vi "HV Rampup.vi"(11 "Ramp Rate":string) -> (3 "standard output":string)   [LabVIEW 2018, in "HV QMH.lvlib"]
uses:
  HV QMH.lvlib
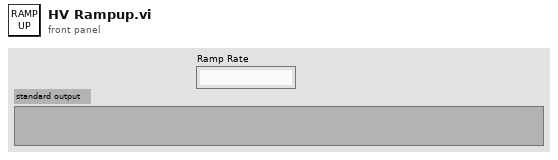
[diagram p1: front panel]
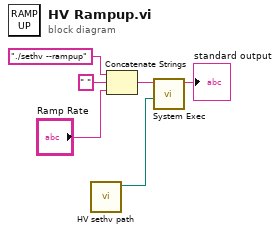
[diagram p0: block diagram]
diagram:
  n1 = call "HV sethv path.vi"() -> ("sethv filepath"=w1:path)  [unwired: 11 in]
  n2 = Concatenate Strings("./sethv --rampup" ("string"), " " ("string"), "Ramp Rate") -> (w3:string)
  n3 = call <vilib>:"System Exec.vi"("working directory"=w1, "command line"=w3) -> ("standard output"=→"standard output":string)  [unwired: 6 in, 3 out]
